vi "Enqueue Message.vi"(8 "error in (no error)":errorcluster, 9 "Message Data":variant, 10 "Message":string, 11 "Process In":refnum<class "Process.lvclass">) -> (0 "error out":errorcluster, 3 "Process Out":refnum<class "Process.lvclass">)   [LabVIEW 2020, in "Process.lvclass"]
doc: "Use the send message VI instead."
uses:
  Process.lvclass
  Process.lvclass/Process.ctl
  Message Cluster.ctl
  Callback/Callback.lvclass
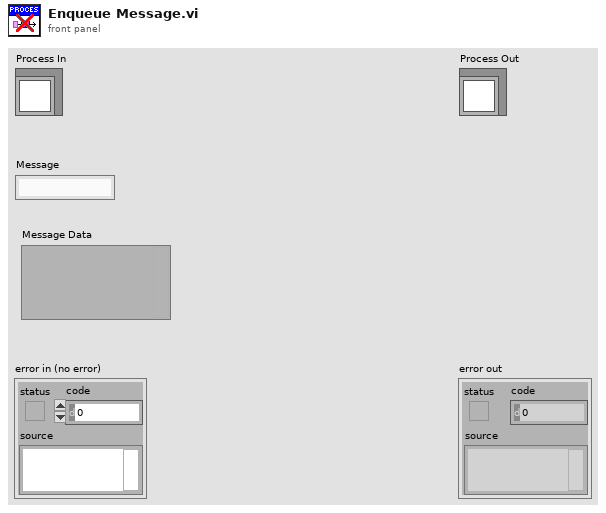
[diagram p1: front panel]
types:
  T1 = enum16{"Send", "Receive", "Request", "Response", "Broadcast"}
  T2 = typedef "Process.lvclass/Message Cluster.ctl" = cluster{"Message":string, "Message Data":variant, "Request Callback":refnum<class "Callback.lvclass">}
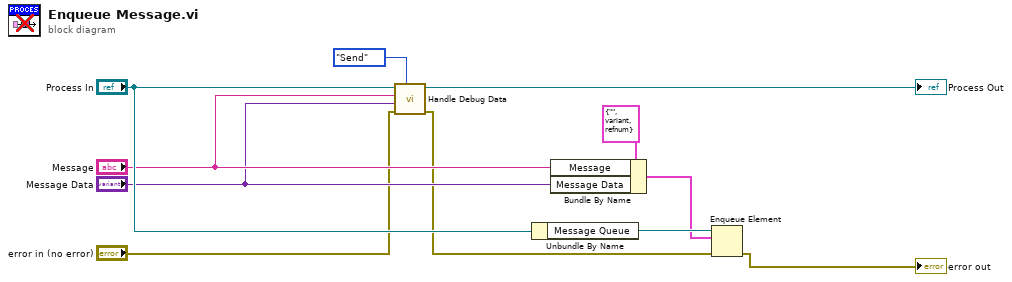
[diagram p0: block diagram]
diagram:
  n1 = call "Handle Debug Data.vi"("Action"=T1."Send", "error in (no error)"="error in (no error)", "Message Data"="Message Data", "Message"="Message", "Process In"="Process In") -> ("error out"=w2:errorcluster, "Process Out"=→"Process Out":refnum<class "Process.lvclass">)  [unwired: 5 in]
  n2 = Unbundle By Name("Process In") -> ("Message Queue"=w9:refnum<queue>)
  n3 = Bundle By Name(cluster=T2 {"Message"="", "Message Data"=variant, "Request Callback"=refnum} ("Message Cluster"), "Message"="Message", "Message Data"="Message Data") -> (w8:T2)
  n4 = Enqueue Element(queue=w9, element=w8, error in (no error)=w2) -> (error out=→"error out":errorcluster)  [unwired: 1 in, 2 out]
